vi "macro_DCMotor_Sim_Execute.vi"() -> ()   [LabVIEW 2019, in "Trajectory_Library.lvlib"]
uses:
  Trajectory_Library.lvlib
  Enum/DCMOTOR_TYPES_ENUM.ctl
  BatterySim_CalculateLoadedBatteryVoltage.vi
panel:
  in  "Motor Dmd (CO)":dbl
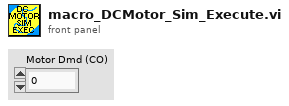
[diagram p1: front panel]
types:
  T1 = typedef "Trajectory_Library.lvlib/DCMOTOR_TYPES_ENUM.ctl" = enum16{"CIM", "AndyMark 9015", "Andy Mark RS 775 125", "Bag", "BaneBots RS 550", "BaneBots RS 775", "Falcon 500", "Mini CIM", "NEO", "NEO 550", "Romi BuiltIn", "Vex 775 Pro", "Snow Blower AM 2235A", "Bosch Seat AM 3493"}
  T2 = typedef "Trajectory_Library.lvlib/LINEAR_SYSTEM_ID_DCMOTOR_MODEL.ctl" = cluster{"DCMOTOR_TYPES":T1, "Num Motors":i32, "Gearing":dbl, "MOI kgm2":dbl}
  T3 = typedef "Trajectory_Library.lvlib/DCMOTOR_SIM_SIMULATION_PARAMS.ctl" = cluster{"Pos Sim Std Dev Rotations":dbl, "Vel Sim Std Dev RPM":dbl}
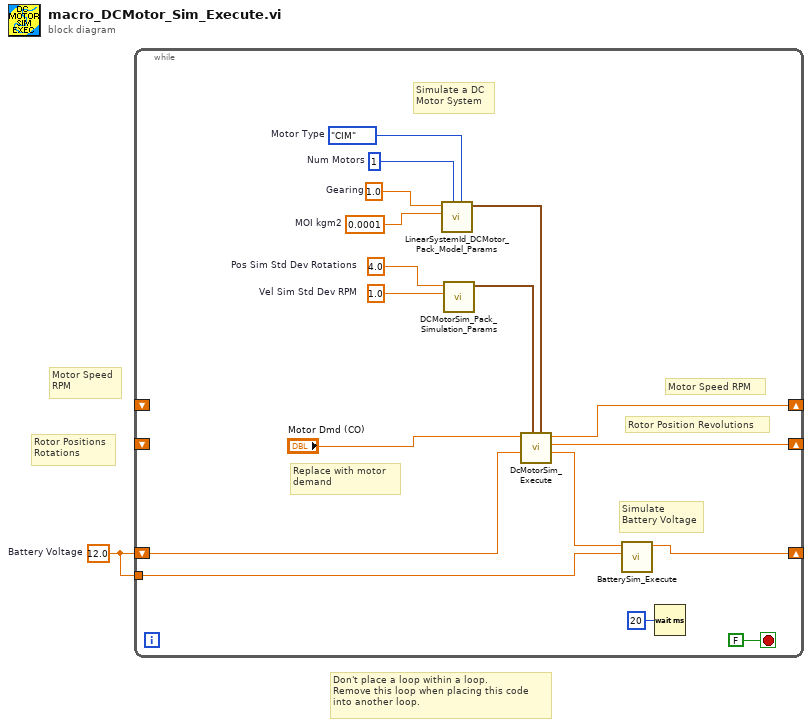
[diagram p0: block diagram]
diagram:
  w1 = 12.0  # Battery Voltage
  # "Rotor Positions\nRotations"
  # "Don't place a loop within a loop. \nRemove this loop when placing this code\ninto another loop."
  # "Motor Speed\nRPM"
  n1 = while {
    shift-right: [w11] -> _
    shift-left: w1 -> [w8]
    shift-right: [w9] -> _
    shift-left: _ -> [_]
    shift-right: [w6] -> _
    shift-left: _ -> [_]
    tunnel: w1 -> [w2]
    stop <- FALSE stop-if-true
    w3 = 4.0  # Pos Sim Std Dev Rotations
    w4 = 1.0  # Vel Sim Std Dev RPM
    w15 = 1.0  # Gearing
    w16 = 0.0001  # MOI kgm2
    w17 = 1  # Num Motors
    w18 = DCMOTOR_TYPES_ENUM."CIM"  # Motor Type
    # "Rotor Position Revolutions"
    # "Motor Speed RPM"
    # "Replace with motor \ndemand"
    # "Simulate\nBattery Voltage"
    # "Simulate a DC \nMotor System"
    n2 = call "LinearSystemId_DCMotor_Pack_Model_Params.vi"("DCMOTOR_TYPES"=w18, "Num Motors"=w17, "MOI kgm2"=w16, "Gearing"=w15) -> ("LinearSystem_ID_DCMotor_Model"=w7:T2)  [unwired: 7 in]
    n3 = call "DCMotorSim_Pack_Simulation_Params.vi"("Vel Sim Std Dev RPM"=w4, "Pos Sim Std Dev Rotations"=w3) -> ("DCMOTOR_Sim_Simulation_Params"=w5:T3)  [unwired: 9 in]
    n4 = call "DcMotorSim_Execute.vi"("DCMotor_Model _Params"=w7, "DCMOTORSim_Simulation_Params"=w5, "Battery Voltage"=w8, "Motor Dmd (CO)"="Motor Dmd (CO)") -> ("Motor Current"=w12:dbl, "Position_Rotations"=w6:dbl, "Velocity_RPM"=w9:dbl)  [unwired: 3 in, 2 out]
    n5 = call "BatterySim_Execute.vi"("Nominal Battery Voltage"=w2, "Current"=w12) -> ("Voltage"=w11:dbl)  [unwired: 9 in]
    n6 = Wait (ms)(milliseconds to wait=u32 20) -> ()  [unwired: 1 out]
  }
